vi "Write Path to check blacklist.vi"(9 "Add to blacklist":string, 11 "CDependencyInspection in":refnum<class "CDependencyInspection.lvclass">) -> (3 "CDependencyInspection out":refnum<class "CDependencyInspection.lvclass">)   [LabVIEW 2020, in "DependencyInspection.lvlib" / "CDependencyInspection.lvclass"]
uses:
  CDependencyInspection.lvclass
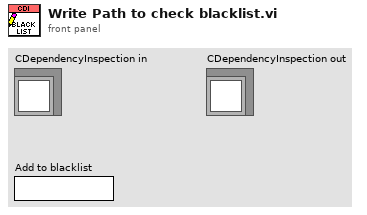
[diagram p1: front panel]
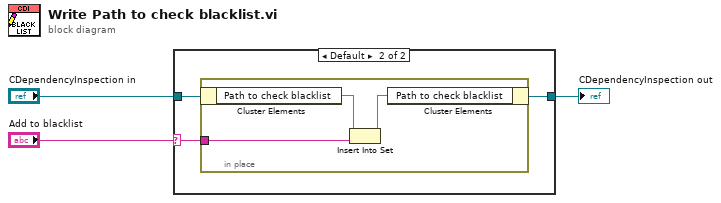
[diagram p0: block diagram]
diagram:
  n1 = case shown="Default" "Add to blacklist" {
    selector: "Add to blacklist" -> [_ w5]
    tunnel: "CDependencyInspection in" -> [w4 w7]
    tunnel: [w4 w6] -> w2
    frame "\u0000" {
    }
    frame Default {
      n2 = in-place {
        in-place-border: w5 -> [w9]
        n3 = in-place-cluster #1(w7) -> ("Path to check blacklist"=w10:set{string})
        n4 = Insert Into Set(10:w9, 11:w10) -> (3:w8:set{string})  [unwired: 1 out]
        n5 = in-place-cluster #1("Path to check blacklist"=w8) -> (w6:refnum<class "CDependencyInspection.lvclass">)
      }
    }
  }
  "CDependencyInspection out" <- w2
